vi "Scanner Update Channels.vi"(10 "Cluster":cluster{"Status":bool, "Channel":T1}, 11 "Control":u8) -> (3 "Numeric":u8)   [LabVIEW 2020, in "Hiden Scanner.lvlib"]
uses:
  Hiden Scanner.lvlib
  Control Channel.ctl
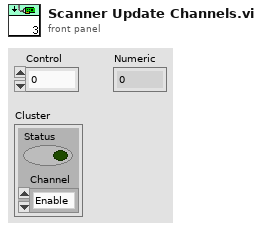
[diagram p1: front panel]
types:
  T1 = typedef "Hiden Scanner.lvlib/Control Channel.ctl" = enum16{"Enable", "Manual Mode", "Jog Up", "Jog Down", "Set Zero Position", "Reset Error", "Move to Pos"}
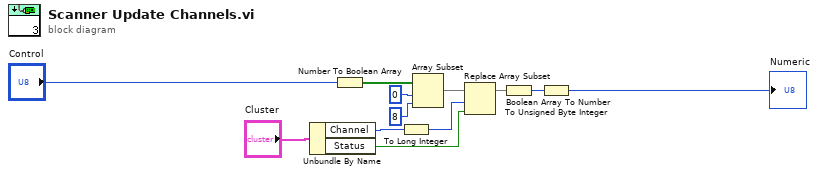
[diagram p0: block diagram]
diagram:
  n1 = Unbundle By Name("Cluster") -> ("Channel"=w5:T1, "Status"=w4:bool)
  n2 = Number To Boolean Array(number="Control") -> (Boolean array=w3:bool[])
  n3 = To Long Integer(number=w5) -> (32bit integer=w6:i32)
  n4 = Array Subset(array=w3, index=0, length=8) -> (w8:bool[])
  n5 = Replace Array Subset(array=w8, new element=w4, index=w6) -> (w7:bool[])
  n6 = Boolean Array To Number(Boolean array=w7) -> (number=w11:u32)
  n7 = To Unsigned Byte Integer(number=w11) -> (unsigned 8bit integer=→"Numeric":u8)
